vi "Decode Tag.vi"(0 "Tag":u32) -> (1 "ID":u32, 2 "Wire Type":T1)   [LabVIEW 2020, in "Protobuf RAW.lvlib"]
uses:
  Protobuf RAW.lvlib
  Type Serializer/Wire Type.ctl
  Wire Type Group/Wire Type Group.lvclass
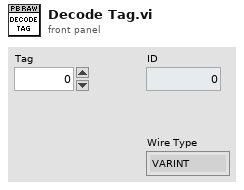
[diagram p1: front panel]
types:
  T1 = typedef "Protobuf RAW.lvlib/Wire Type Group.lvclass/Wire Type.ctl" = enum16{"VARINT", "I64", "LEN", "SGROUP", "EGROUP", "I32"}
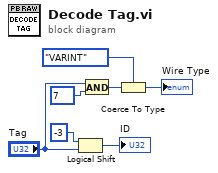
[diagram p0: block diagram]
diagram:
  n1 = Logical Shift(y=i16 -3, x="Tag") -> (x << y=→"ID":u32)
  n2 = And(x="Tag", y=u64 7 ("Tag")) -> (x .and. y?=w5:u64)
  n3 = Coerce To Type(0:w5, 1:Wire_Type."VARINT" ("Wire Type")) -> (2:→"Wire Type":T1)
